vi "Send Message to Launcher.vi"(8 "error in (no error)":errorcluster, 10 "Msg to Launcher":string, 11 "Actor wLauncher in":refnum<class "Actor wLauncher.lvclass">) -> (0 "error out":errorcluster, 3 "Actor wLauncher out":refnum<class "Actor wLauncher.lvclass">)   [LabVIEW 2017, in "Framework.lvlib" / "Actor wLauncher.lvclass"]
uses:
  Actor wLauncher.lvclass
  Actor wLauncher.lvclass/Actor wLauncher.ctl
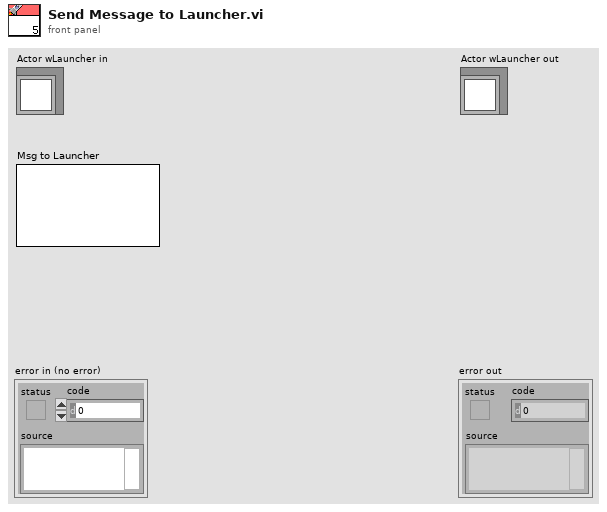
[diagram p1: front panel]
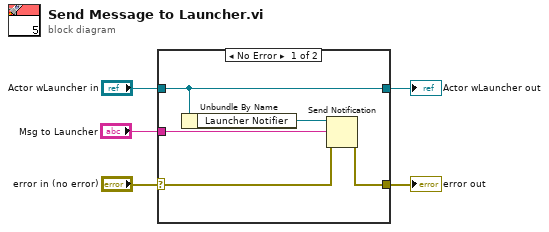
[diagram p0: block diagram]
diagram:
  n1 = case shown="No Error" "error in (no error)" {
    selector: "error in (no error)" -> [w8 w12]
    tunnel: [w7 w12] -> w4
    tunnel: [w10 w11] -> w2
    tunnel: "Actor wLauncher in" -> [w10 w11]
    tunnel: "Msg to Launcher" -> [w6 _]
    frame No Error {
      n2 = Unbundle By Name(w10) -> ("Launcher Notifier"=w9:refnum<notifier>)
      n3 = Send Notification(notification=w6, notifier=w9, error in (no error)=w8) -> (error out=w7:errorcluster)  [unwired: 1 out]
    }
    frame Error {
    }
  }
  "error out" <- w4
  "Actor wLauncher out" <- w2
